vi "Connect Terminals.vi"(6 "Auto Route? (F)":bool, 7 "Auto Wire? (T)":bool, 8 "Error In":errorcluster, 9 "Source Terminal":refnum<vi>, 11 "Sink Terminal":refnum<vi>) -> (0 "Error Out":errorcluster)   [LabVIEW 2019, in "gRPC Template Creation Utility.lvlib"]
uses:
  gRPC Template Creation Utility.lvlib
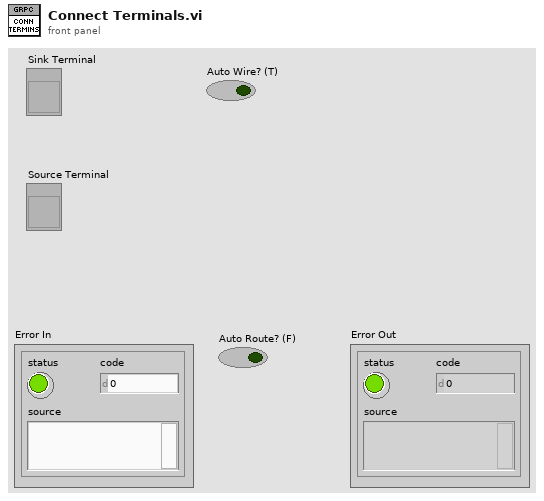
[diagram p1: front panel]
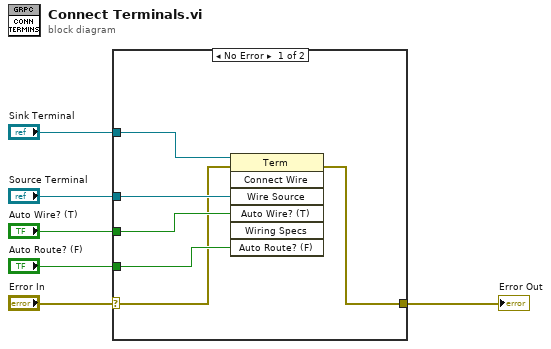
[diagram p0: block diagram]
diagram:
  n1 = case shown="No Error" "Error In" {
    selector: "Error In" -> [w7 w13]
    tunnel: "Source Terminal" -> [w12 _]
    tunnel: [w11 w13] -> w4
    tunnel: "Auto Wire? (T)" -> [w10 _]
    tunnel: "Auto Route? (F)" -> [w9 _]
    tunnel: "Sink Terminal" -> [w8 _]
    frame No Error {
      n2 = invoke class="Term" method="Connect Wire"(reference=w8, error in=w7, "Wire Source"=w12, "Auto Wire? (T)"=w10, "Auto Route? (F)"=w9) -> (error out=w11:errorcluster)  [unwired: 2 in, 6 out]
    }
    frame Error {
    }
  }
  "Error Out" <- w4
